vi "Display on Menu - Action.vi"(4 "Update Menu (T)":bool=TRUE, 5 "Item Tag":string, 6 "Previous Active Display":u16, 7 "Active Display":u16, 8 "error in":errorcluster, 9 "MenuRef":refnum<k9>, 10 "FP Bounds":T1={"Left"=105, "Top"=-7, "Right"=1816, "Bottom"=994}, 11 "VI Ref":refnum<vi>) -> (0 "error out":errorcluster, 3 "VI Ref":refnum<vi>)   [LabVIEW 2014]
uses:
  <vilib>/Utility/miscctls.llb/LVRectTypeDef.ctl
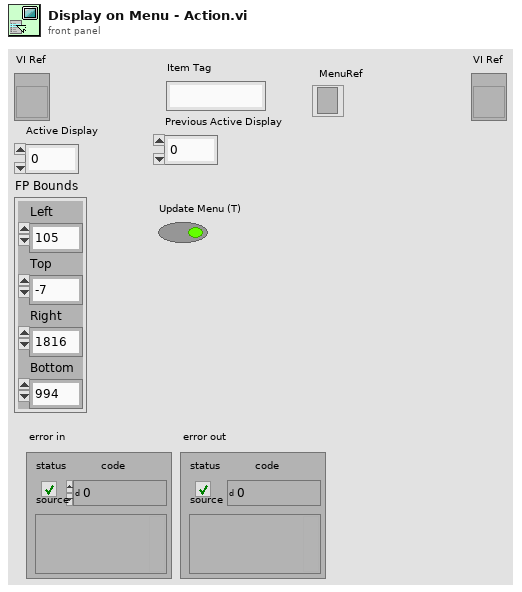
[diagram p1: front panel]
types:
  T1 = typedef "LVRectTypeDef.ctl" = cluster{"Left":i16, "Top":i16, "Right":i16, "Bottom":i16}
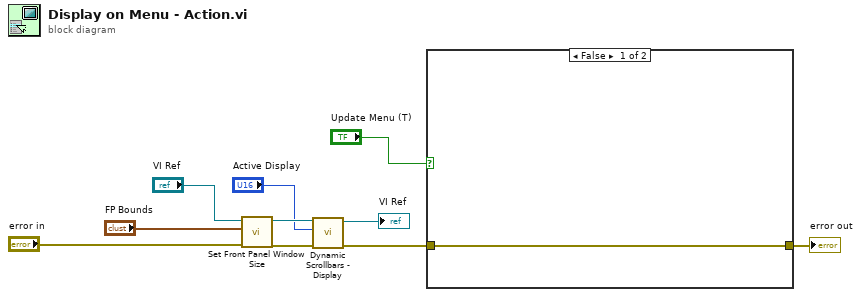
[diagram p0: block diagram]
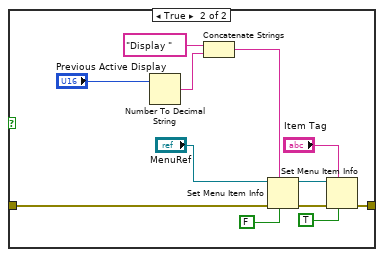
[diagram p2: hidden frame]
diagram:
  n1 = call "Set Front Panel Window Size.vi"("error in"="error in", "Front Panel Window:Window Bounds"="FP Bounds", "VI Ref"="VI Ref") -> ("error out"=w10:errorcluster, "VI Ref"=w9:refnum<vi>)  [unwired: 7 in]
  n2 = call "Dynamic Scrollbars - Display.vi"("error in"=w10, "Active Display in"="Active Display", "VI Ref"=w9) -> ("error out"=w4:errorcluster, "VI Ref"=→"VI Ref":refnum<vi>)  [unwired: 6 in, 1 out]
  n3 = case shown="False" "Update Menu (T)" {
    tunnel: w4 -> [w11 w14]
    tunnel: [w11 w12] -> w3
    frame False {
    }
    frame True {
      n4 = Number To Decimal String(number="Previous Active Display") -> (decimal integer string=w18:string)  [unwired: 1 in]
      n5 = Concatenate Strings("Display ", w18) -> (w17:string)
      n6 = Set Menu Item Info(6:FALSE ("checked"), 7:w17, 8:w14, 11:"MenuRef") -> (0:w23:errorcluster, 3:w22:refnum<k9>)  [unwired: 3 in]
      n7 = Set Menu Item Info(6:TRUE ("checked"), 7:"Item Tag", 8:w23, 11:w22) -> (0:w12:errorcluster)  [unwired: 3 in, 1 out]
    }
  }
  "error out" <- w3
